vi "Update DAQ Device Name.vi"(9 "Device Name":string, 11 "Lines in (String)":string) -> (3 "Lines out (DAQmx Physical Channels)":tag)   [LabVIEW 2015]
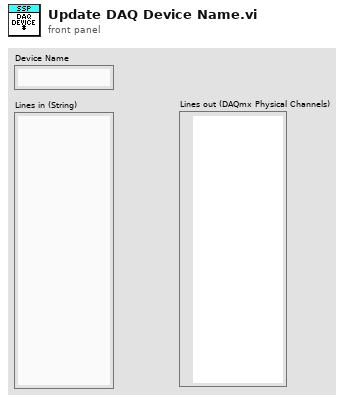
[diagram p1: front panel]
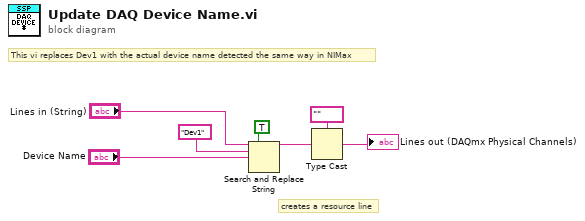
[diagram p0: block diagram]
diagram:
  # "creates a resource line"
  # "This vi replaces Dev1 with the actual device name detected the same way in NIMax"
  n1 = Search and Replace String(replace all?=TRUE ("replace all? (F)"), input string="Lines in (String)", search string="Dev1", replace string="Device Name") -> (result string=w4:string)  [unwired: 4 in, 3 out]
  n2 = Type Cast(type=tag "" ("lines"), x=w4) -> (*(type *) &x=→"Lines out (DAQmx Physical Channels)":tag)
